vi "euler_to_rotation.vi"(11 "Theta XYZ":dbl[](array[numeric])) -> (3 "Rotation":T1)   [LabVIEW 2013]
uses:
  <vilib>/Analysis/Matrix/Datatypes/RealMatrix.ctl
  <vilib>/Analysis/baseanly.llb/Real A x B.vi
  <vilib>/Analysis/Matrix/NI_Matrix.lvlib
  <vilib>/Analysis/NI_AALBase.lvlib
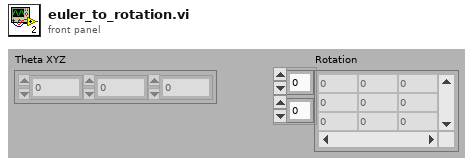
[diagram p1: front panel]
types:
  T1 = typedef "NI_Matrix.lvlib/RealMatrix.ctl" = dbl[][]
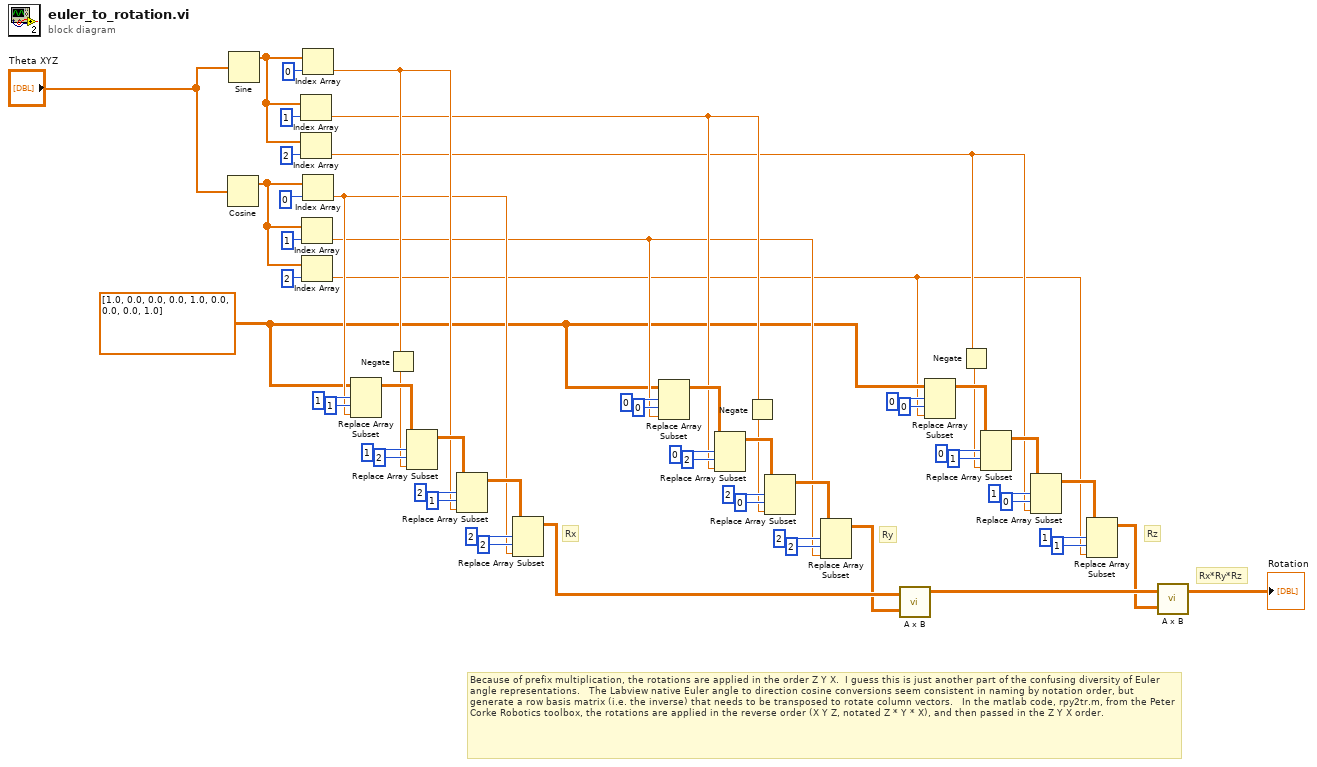
[diagram p0: block diagram]
diagram:
  w9 = T1 [[1.0, 0.0, 0.0], [0.0, 1.0, 0.0], [0.0, 0.0, 1.0]] ("A + B")
  # "Because of prefix multiplication, the rotations are applied in the order Z Y X.  I guess this is just another part of the confusing diversity of Euler angle representations.   The Labview native Euler angle to direction cosine conversions seem consistent in naming by notation order, but generate a row basis matrix (i.e. the inverse) that needs to be transposed to rotate column vectors.   In the matlab code, rpy2tr.m, from the Peter Corke Robotics toolbox, the rotations are applied in the reverse order (X Y Z, notated Z * Y * X), and then passed in the Z Y X order."
  # "Rx*Ry*Rz"
  # "Rz"
  # "Ry"
  # "Rx"
  n1 = Cosine(x="Theta XYZ") -> (cos(x)=w49:dbl[])
  n2 = Sine(x="Theta XYZ") -> (sin(x)=w53:dbl[])
  n3 = Index Array(array=w53, index=1) -> (element=w23:dbl)
  n4 = Index Array(array=w53, index=2) -> (element=w7:dbl)
  n5 = Index Array(array=w49, index=1) -> (element=w21:dbl)
  n6 = Index Array(array=w49, index=2) -> (element=w6:dbl)
  n7 = Index Array(array=w53, index=0) -> (element=w36:dbl)
  n8 = Index Array(array=w49, index=0) -> (element=w35:dbl)
  n9 = Replace Array Subset(array=w9, new element=w35, index (row)=1, index (col)=1) -> (w46:T1)
  n10 = Negate(x=w36) -> (-x=w37:dbl)
  n11 = Replace Array Subset(array=w46, new element=w37, index (row)=1, index (col)=2) -> (w45:T1)
  n12 = Replace Array Subset(array=w45, new element=w36, index (row)=2, index (col)=1) -> (w44:T1)
  n13 = Replace Array Subset(array=w44, new element=w35, index (row)=2, index (col)=2) -> (w5:T1)
  n14 = Replace Array Subset(array=w9, new element=w21, index (row)=0, index (col)=0) -> (w32:T1)
  n15 = Replace Array Subset(array=w32, new element=w23, index (row)=0, index (col)=2) -> (w31:T1)
  n16 = Negate(x=w23) -> (-x=w22:dbl)
  n17 = Replace Array Subset(array=w31, new element=w22, index (row)=2, index (col)=0) -> (w30:T1)
  n18 = Replace Array Subset(array=w30, new element=w21, index (row)=2, index (col)=2) -> (w4:T1)
  n19 = call-poly <vilib>:"A x B.vi"("B"=w4, "A"=w5) -> ("A x B"=w3:T1)  [unwired: 1 out]
  n20 = Replace Array Subset(array=w9, new element=w6, index (row)=0, index (col)=0) -> (w18:T1)
  n21 = Negate(x=w7) -> (-x=w8:dbl)
  n22 = Replace Array Subset(array=w18, new element=w8, index (row)=0, index (col)=1) -> (w17:T1)
  n23 = Replace Array Subset(array=w17, new element=w7, index (row)=1, index (col)=0) -> (w16:T1)
  n24 = Replace Array Subset(array=w16, new element=w6, index (row)=1, index (col)=1) -> (w2:T1)
  n25 = call-poly <vilib>:"A x B.vi"("B"=w2, "A"=w3) -> ("A x B"=→"Rotation":T1)  [unwired: 1 out]
